vi "kim-read file -one.vi"(0 "File Path Control":path, 6 "Numeric Control":i32, 7 "plot type":T3(ring)=enum."plot vs Temperature", 8 "container action":T4) -> (11 "Plot linew":T1, 13 "Plot freq":T2, 14 "OK?":bool, 15 "Temperature (K) Array":dbl[](array[numeric]), 16 "time (min) array":dbl[](array[numeric]), 17 "Field (T) Array":dbl[](array[numeric]), 18 "Gamma (kHz) Array":dbl[](array[numeric]), 19 "Frequency (kHz) Array":dbl[](array[numeric]))   [LabVIEW 2015]
uses:
  container action.ctl
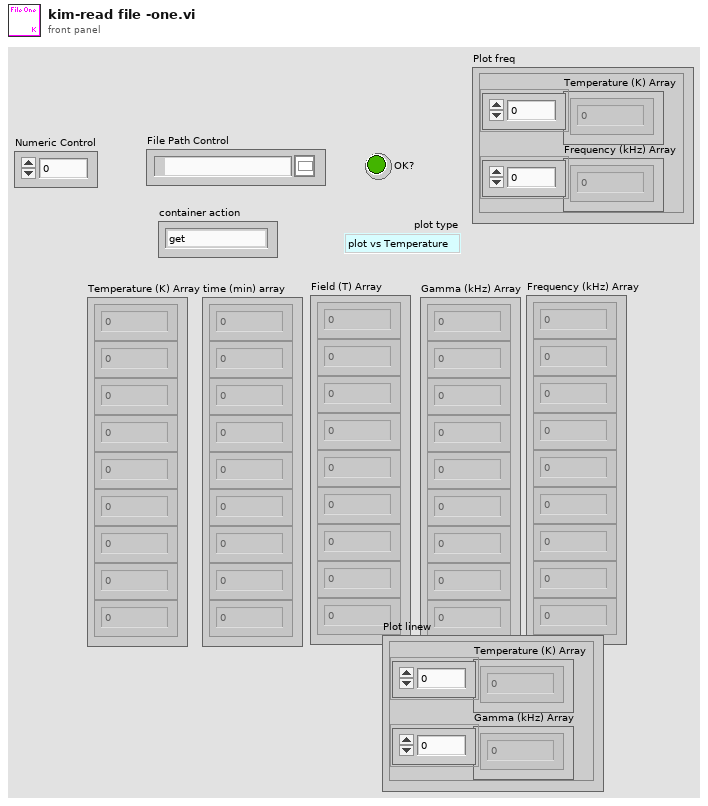
[diagram p1: front panel]
types:
  T1 = cluster{"Temperature (K) Array":dbl[], "Gamma (kHz) Array":dbl[]}
  T2 = cluster{"Temperature (K) Array":dbl[], "Frequency (kHz) Array":dbl[]}
  T3 = enum16{"plot vs Magnetic Field", "plot vs Temperature"}
  T4 = typedef "container action.ctl" = enum16{"get", "read file", "plot", "init", "set"}
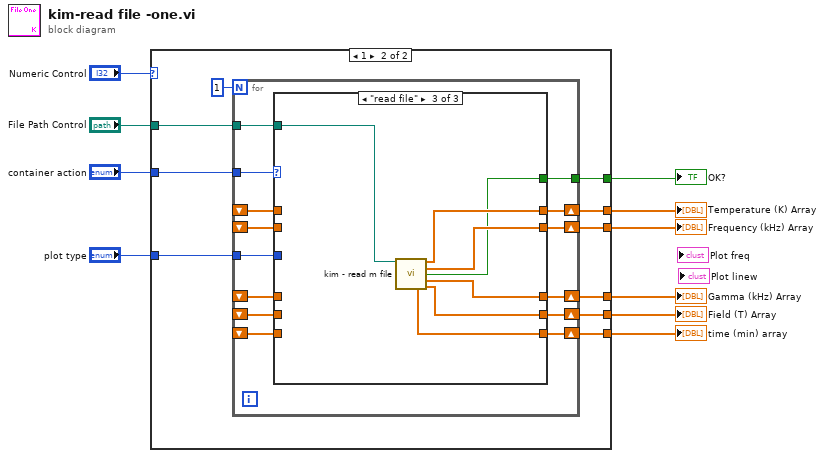
[diagram p0: block diagram]
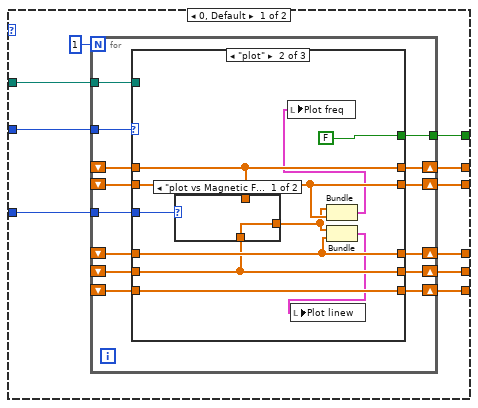
[diagram p2: hidden frame]
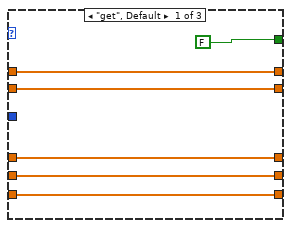
[diagram p3: hidden frame]
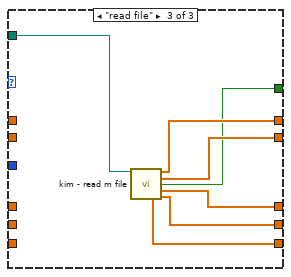
[diagram p5: hidden frame]
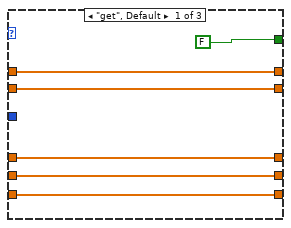
[diagram p6: hidden frame]
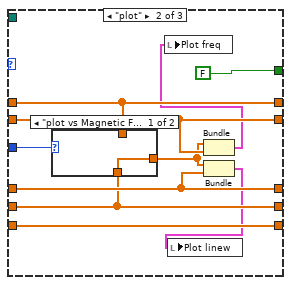
[diagram p7: hidden frame]
diagram:
  n1 = case shown="1" "Numeric Control" {
    tunnel: [w20 w69] -> w10
    tunnel: [w19 w68] -> w9
    tunnel: [w18 w67] -> w8
    tunnel: [w17 w66] -> w7
    tunnel: [w12 w61] -> w3
    tunnel: [w16 w65] -> w6
    tunnel: "File Path Control" -> [w14 w63]
    tunnel: "container action" -> [w13 w62]
    tunnel: "plot type" -> [w11 w60]
    frame 0, Default {
      n2 = for {
        N: 1 -> [_]
        shift-right: [w30] -> w16
        shift-left: _ -> [w25]
        shift-right: [w31] -> w17
        shift-left: _ -> [w26]
        shift-right: [w32] -> w18
        shift-left: _ -> [w27]
        shift-right: [w33] -> w19
        shift-left: _ -> [w28]
        shift-right: [w34] -> w20
        shift-left: _ -> [w29]
        tunnel: w14 -> [w24]
        tunnel: w13 -> [w23]
        tunnel: [w22] -> w12
        tunnel: w11 -> [w21]
        n3 = case shown="\"plot\"" w23 {
          tunnel: [w40 w43 w59] -> w34
          tunnel: [w39 w48 w58] -> w33
          tunnel: [w38 w47 w57] -> w32
          tunnel: [w37 w44 w56] -> w31
          tunnel: [FALSE FALSE w53] -> w22
          tunnel: [w36 w50 w55] -> w30
          tunnel: w24 -> [_ _ w54]
          tunnel: w29 -> [w40 w43 _]
          tunnel: w28 -> [w39 w48 _]
          tunnel: w27 -> [w38 w47 _]
          tunnel: w26 -> [w37 w44 _]
          tunnel: w25 -> [w36 w50 _]
          tunnel: w21 -> [_ w46 _]
          frame "get", Default {
          }
          frame "plot" {
            n4 = case shown="\"plot vs Magnetic Field\", Default" w46 {
              tunnel: [w51 w52] -> w45
              tunnel: w44 -> [w51 _]
              tunnel: w43 -> [_ w52]
              frame "plot vs Magnetic Field", Default {
              }
              frame "plot vs Temperature" {
              }
            }
            n5 = Bundle("Temperature (K) Array"=w45, "Frequency (kHz) Array"=w48) -> (w42:T2)  [unwired: 1 in]
            n6 = local write "Plot freq"(w42) -> ()
            n7 = Bundle("Temperature (K) Array"=w45, "Gamma (kHz) Array"=w47) -> (w41:T1)  [unwired: 1 in]
            n8 = local write "Plot linew"(w41) -> ()
          }
          frame "read file" {
            n9 = call "kim - read m file.vi"("file path"=w54) -> ("Temperature (K) Array"=w59:dbl[], "Frequency (kHz) Array"=w58:dbl[], "OK?"=w53:bool, "Gamma (kHz) Array"=w57:dbl[], "time (min)"=w55:dbl[], "Field (T) Array"=w56:dbl[])  [unwired: 9 in]
          }
        }
      }
    }
    frame 1 {
      n10 = for {
        N: 1 -> [_]
        shift-right: [w79] -> w65
        shift-left: _ -> [w74]
        shift-right: [w80] -> w66
        shift-left: _ -> [w75]
        shift-right: [w81] -> w67
        shift-left: _ -> [w76]
        shift-right: [w82] -> w68
        shift-left: _ -> [w77]
        shift-right: [w83] -> w69
        shift-left: _ -> [w78]
        tunnel: w63 -> [w73]
        tunnel: w62 -> [w72]
        tunnel: [w71] -> w61
        tunnel: w60 -> [w70]
        n11 = case shown="\"read file\"" w72 {
          tunnel: [w89 w92 w108] -> w83
          tunnel: [w88 w97 w107] -> w82
          tunnel: [w87 w96 w106] -> w81
          tunnel: [w86 w93 w105] -> w80
          tunnel: [FALSE FALSE w102] -> w71
          tunnel: [w85 w99 w104] -> w79
          tunnel: w73 -> [_ _ w103]
          tunnel: w78 -> [w89 w92 _]
          tunnel: w77 -> [w88 w97 _]
          tunnel: w76 -> [w87 w96 _]
          tunnel: w75 -> [w86 w93 _]
          tunnel: w74 -> [w85 w99 _]
          tunnel: w70 -> [_ w95 _]
          frame "get", Default {
          }
          frame "plot" {
            n12 = case shown="\"plot vs Magnetic Field\", Default" w95 {
              tunnel: [w100 w101] -> w94
              tunnel: w93 -> [w100 _]
              tunnel: w92 -> [_ w101]
              frame "plot vs Magnetic Field", Default {
              }
              frame "plot vs Temperature" {
              }
            }
            n13 = Bundle("Temperature (K) Array"=w94, "Frequency (kHz) Array"=w97) -> (w91:T2)  [unwired: 1 in]
            n14 = local write "Plot freq"(w91) -> ()
            n15 = Bundle("Temperature (K) Array"=w94, "Gamma (kHz) Array"=w96) -> (w90:T1)  [unwired: 1 in]
            n16 = local write "Plot linew"(w90) -> ()
          }
          frame "read file" {
            n17 = call "kim - read m file.vi"("file path"=w103) -> ("Temperature (K) Array"=w108:dbl[], "Frequency (kHz) Array"=w107:dbl[], "OK?"=w102:bool, "Gamma (kHz) Array"=w106:dbl[], "time (min)"=w104:dbl[], "Field (T) Array"=w105:dbl[])  [unwired: 9 in]
          }
        }
      }
    }
  }
  "time (min) array" <- w6
  "Field (T) Array" <- w7
  "Gamma (kHz) Array" <- w8
  "Frequency (kHz) Array" <- w9
  "Temperature (K) Array" <- w10
  "OK?" <- w3
